vi "register.public_dir_lua.vi"(5 "LuaVIEW reference":T1) -> (15 "error out":errorcluster)   [LabVIEW 2012]
doc: "Tries to register all VIs ending in \"_lua.vi\" in a directory and, recursively, in any subdirectories or llbs, or inside a built executable, with the public function registry. The directory path can be absolute or relative to the resource base path. The functions in the public registry are set when a virtual machine is instantiated. Thus, the registered functions will be available to subsequently opened LuaVIEW states yet remain invisible to already running scripts (including the script that called this registration function). The registered functions remain loaded until the public registry is cleaned up.\nParameters:\nstr:dirpath, path of a directory holding function VIs.\nErrors:\nDirectory path invalid.\nFunction name invalid.\nFunction improperly documented.\nCould not load function VI.\nFunction VI has an invalid connector pane."
uses:
  typedefs/t_LuaVIEW Reference.ctl
  subvis/private/LuaVIEW Pull (path).vi
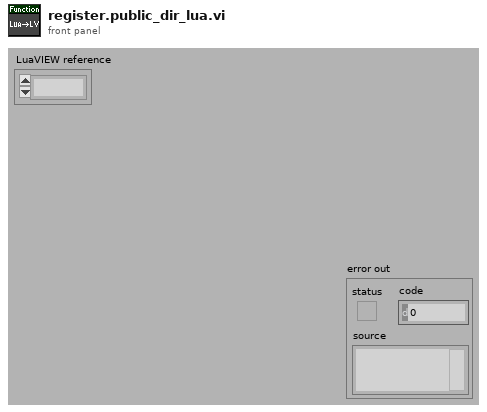
[diagram p1: front panel]
types:
  T1 = typedef "t_LuaVIEW Reference.ctl" = refnum<k1>
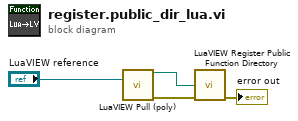
[diagram p0: block diagram]
diagram:
  n1 = call-poly "LuaVIEW Pull (poly).vi"("LuaVIEW reference in"="LuaVIEW reference") -> ("path"=w1:path, "error out"=w3:errorcluster)  [unwired: 12 in, 1 out]
  n2 = call "LuaVIEW Register Public Function Directory.vi"("base path"=w1, "error in (no error)"=w3) -> ("error out"=→"error out":errorcluster)  [unwired: 13 in]
